vi "开启关闭最值.vi"(3 "计算参数 in":T1, 5 "Array in":dbl[](array[numeric])) -> (0 "计算参数 out":T1, 2 "Array out":dbl[](array[numeric]))   [LabVIEW 2013]
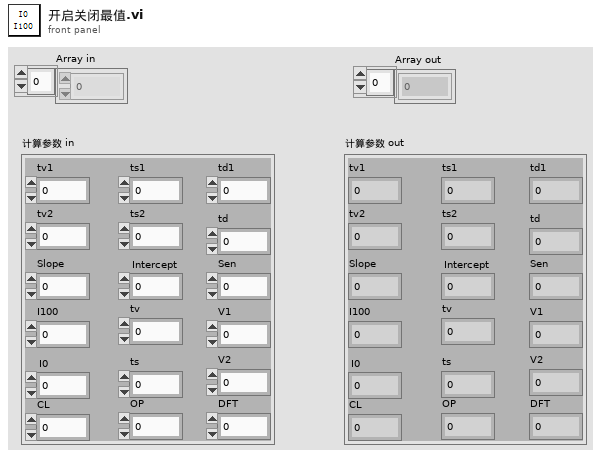
[diagram p1: front panel]
types:
  T1 = cluster{"tv1":dbl, "tv2":dbl, "tv":dbl, "ts1":dbl, "ts2":dbl, "ts":dbl, "td1":dbl, "td":dbl, "Slope":dbl, "Intercept":dbl, "I100":dbl, "I0":dbl, "Sen":dbl, "V1":dbl, "V2":dbl, "CL":dbl, "OP":dbl, "DFT":dbl}
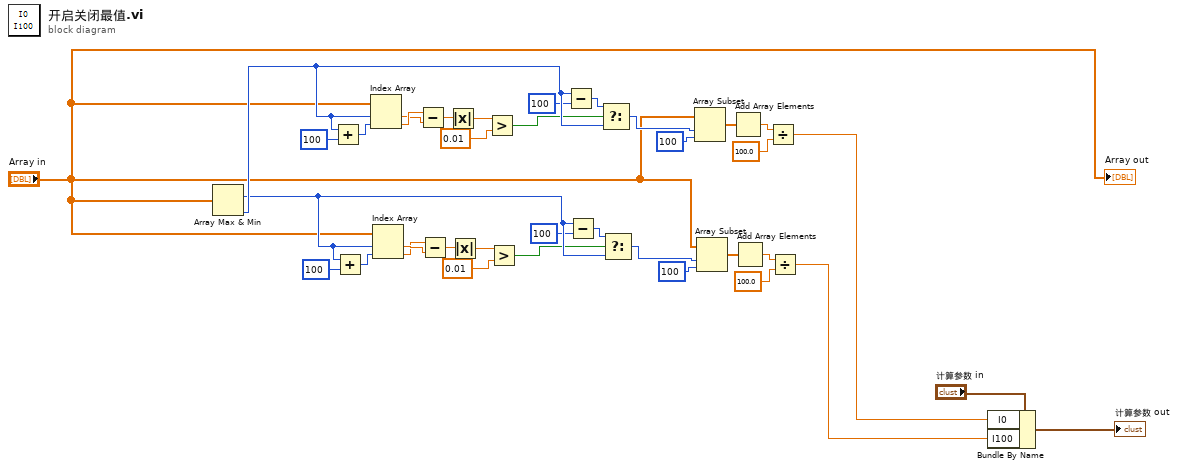
[diagram p0: block diagram]
diagram:
  n1 = Array Max & Min(array="Array in") -> (max index (indices)=w20:i32, min index (indices)=w36:i32)  [unwired: 2 out]
  n2 = Add(x=w36, y=100) -> (x+y=w35:i32)
  n3 = Add(x=w20, y=100) -> (x+y=w5:i32)
  n4 = Index Array(array="Array in", index #1=w36, index #2=w35) -> (element #1=w32:dbl, element #2=w33:dbl)
  n5 = Index Array(array="Array in", index #1=w20, index #2=w5) -> (element #1=w8:dbl, element #2=w7:dbl)
  n6 = Subtract(x=w33, y=w32) -> (x-y=w31:dbl)
  n7 = Subtract(x=w7, y=w8) -> (x-y=w9:dbl)
  n8 = Absolute Value(x=w31) -> (abs(x)=w30:dbl)
  n9 = Absolute Value(x=w9) -> (abs(x)=w10:dbl)
  n10 = Greater?(x=w30, y=0.01) -> (0:w23:bool)
  n11 = Greater?(x=w10, y=0.01) -> (0:w17:bool)
  n12 = Subtract(x=w36, y=100) -> (x-y=w22:i32)
  n13 = Subtract(x=w20, y=100) -> (x-y=w18:i32)
  n14 = Select(t=w22, s=w23, f=w36) -> (s? t:f=w21:i32)
  n15 = Select(t=w18, s=w17, f=w20) -> (s? t:f=w19:i32)
  n16 = Array Subset(array="Array in", index=w21, length=100 ("长度")) -> (w27:dbl[])
  n17 = Array Subset(array="Array in", index=w19, length=100 ("长度")) -> (w13:dbl[])
  n18 = Add Array Elements(numeric array=w27) -> (sum=w26:dbl)
  n19 = Add Array Elements(numeric array=w13) -> (sum=w14:dbl)
  n20 = Divide(x=w26, y=100.0) -> (x/y=w4:dbl)
  n21 = Divide(x=w14, y=100.0) -> (x/y=w3:dbl)
  n22 = Bundle By Name(cluster="计算参数 in", "I0"=w4, "I100"=w3) -> (→"计算参数 out":T1)
  "Array out" <- "Array in"
